vi "Init.vi"(8 "error in":errorcluster, 11 "Simulated CANopen Node in":refnum<class "Simulated CANopen Node.lvclass">) -> (0 "error out":errorcluster, 3 "Simulated CANopen Node out":refnum<class "Simulated CANopen Node.lvclass">)   [LabVIEW 2020, in "Simulated CANopen Node.lvclass"]
uses:
  Simulated CANopen Node.lvclass
  Simulated CANopen Node.lvclass/Simulated CANopen Node.ctl
  HAL/Source/Interfaces/IMessage/IMessage.lvclass
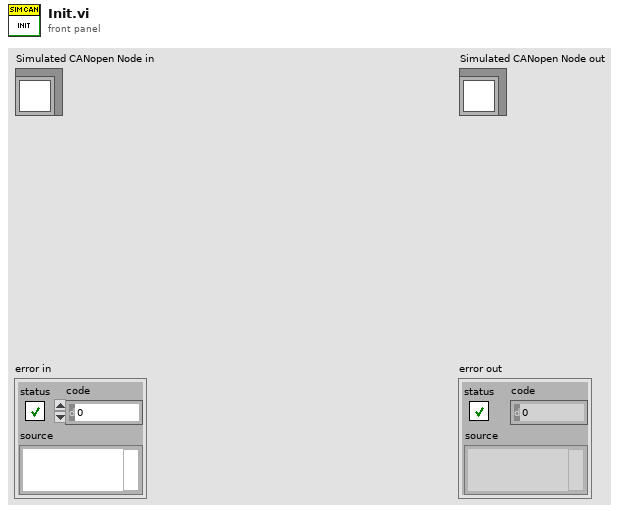
[diagram p1: front panel]
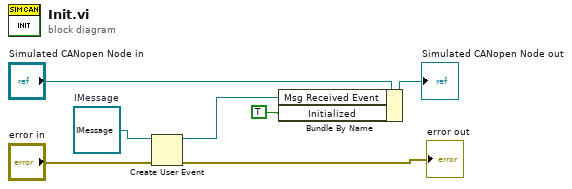
[diagram p0: block diagram]
diagram:
  w3 = refnum<class "IMessage.lvclass"> refnum  # IMessage
  n1 = Create User Event(user event datatype=w3, error in="error in") -> (user event=w2:refnum<user-event>, error out=→"error out":errorcluster)
  n2 = Bundle By Name(cluster="Simulated CANopen Node in", "Msg Received Event"=w2, "Initialized"=TRUE) -> (→"Simulated CANopen Node out":refnum<class "Simulated CANopen Node.lvclass">)
